vi "CylinderWork.vi"(8 "error in (no error)":errorcluster, 11 "TestBench in":refnum<class "TestBench.lvclass">) -> (0 "error out":errorcluster, 3 "TestBench out":refnum<class "TestBench.lvclass">)   [LabVIEW 2019, in "TestBench.lvlib" / "TestBench.lvclass"]
uses:
  TestBench.lvclass
  TestBench.lvclass/TestBench.ctl
  SignalProcessing/SignalProcessing Messages/ActorEventMessage Msg/ActorEventMessage Msg.lvclass/ActorEventMessage Msg.ctl
  <vilib>/ActorFramework/Message Enqueuer/Message Enqueuer.lvclass/Message Enqueuer.ctl
  <vilib>/ActorFramework/Message Enqueuer/Enqueue.vi
  SignalProcessing/SignalProcessing Messages/ActorEventMessage Msg/ActorEventMessage Msg.lvclass
  C:/Program Files (x86)/National Instruments/LabVIEW 2019/vi.lib/ActorFramework/Message/Message.lvclass
  <vilib>/ActorFramework/Message Priority Queue/Priority Enqueue.vi
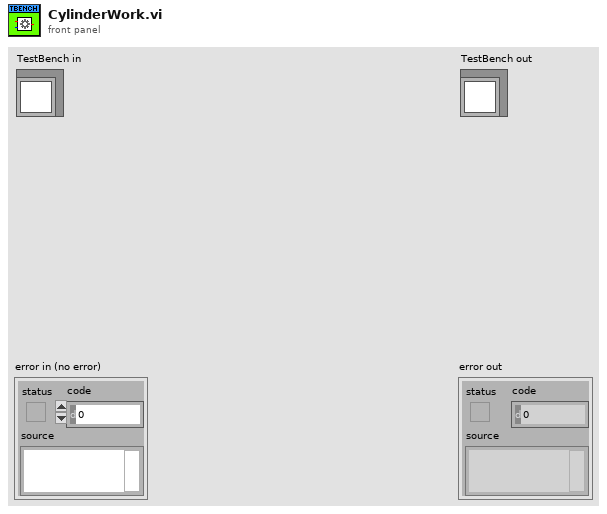
[diagram p1: front panel]
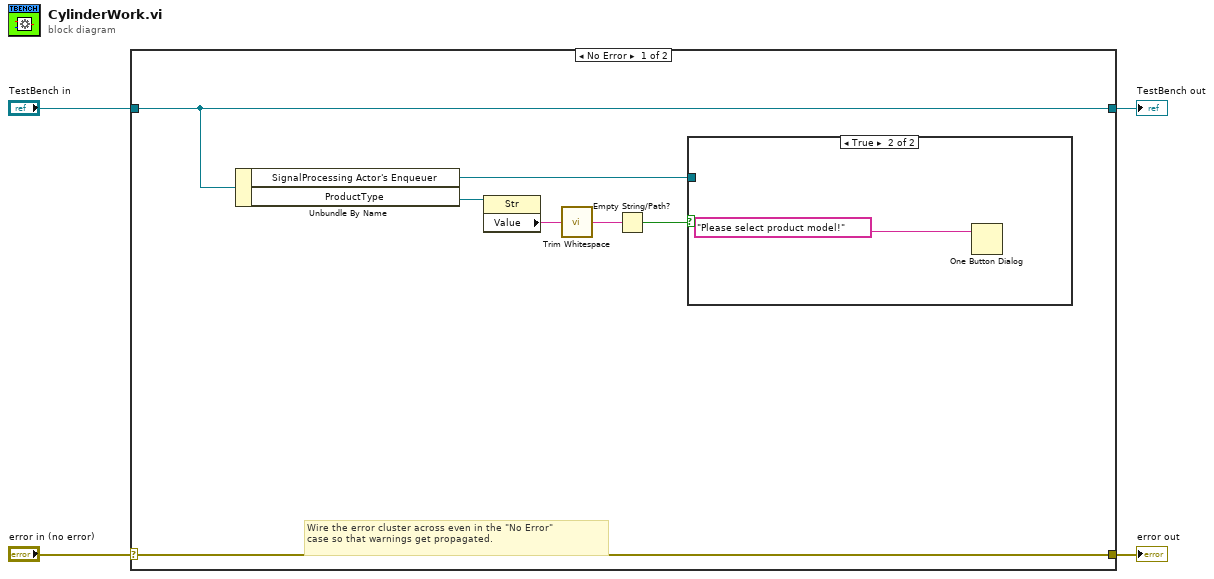
[diagram p0: block diagram]
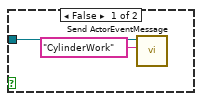
[diagram p2: hidden frame]
diagram:
  n1 = case shown="No Error" "error in (no error)" {
    selector: "error in (no error)" -> [w11 w16]
    tunnel: [w11 w16] -> w3
    tunnel: [w10 w15] -> w1
    tunnel: "TestBench in" -> [w10 w15]
    frame No Error {
      # "Wire the error cluster across even in the \"No Error\"\ncase so that warnings get propagated."
      n2 = Unbundle By Name(w10) -> ("SignalProcessing Actor's Enqueuer"=w6:refnum<class "Message Enqueuer.lvclass">, "ProductType"=w9:refnum<vi>)
      n3 = property class="Str"(reference=w9) -> ("Value"=w8:string)  [unwired: 1 in, 2 out]
      n4 = call <vilib>:"Trim Whitespace.vi"("string"=w8) -> ("trimmed string"=w7:string)  [unwired: 1 in]
      n5 = Empty String/Path?(string/path=w7) -> (empty?=w5:bool)
      n6 = case shown="True" w5 {
        tunnel: w6 -> [w13 _]
        frame False {
          n7 = call "Send ActorEventMessage.vi"("EventMessage"="CylinderWork", "Message Enqueuer"=w13) -> ()  [unwired: 8 in, 2 out]
        }
        frame True {
          n8 = One Button Dialog(message="Please select product model!") -> ()  [unwired: 1 in, 1 out]
        }
      }
    }
    frame Error {
    }
  }
  "error out" <- w3
  "TestBench out" <- w1
